vi "SNEdit.vi"() -> ()   [LabVIEW 2011]
uses:
  data/VCI_CAN.dll
panel:
  in  "devtype":u16(ring)=2 caption="设备类型：" items=["USB-CAN"=2, "USB-CAN2.0"=3]
  in  "snedit":bool
  in  "close":bool
  in  "open":bool
  out "canopen":bool caption="设备打开："
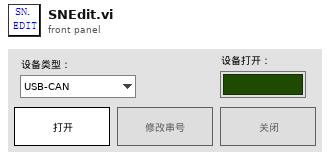
[diagram p1: front panel]
types:
  T1 = enum16{"Init", "EventReg", "Run", "Release", "Exit"}
  T2 = cluster{"hw_Version":u16, "fw_Version":u16, "dr_Version":u16, "in_Version":u16, "irq_Num":u16, "can_Num":u8, "str_Serial_Num":string, "str_hw_Type":string, "Reserved":u8[]}
  T3 = cluster{"hw_Version":u16, "fw_Version":u16, "dr_Version":u16, "in_Version":u16, "irq_Num":u16, "can_Num":u8, "reserved":u8, "str_Serial_Num":string, "str_hw_Type":string, "str_GYUsb_Serial":string[]}
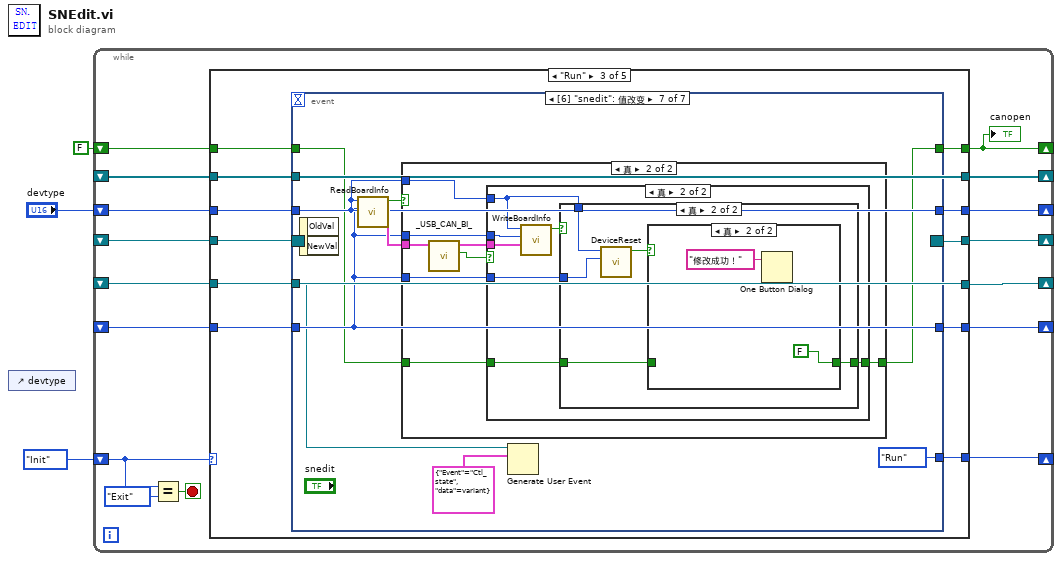
[diagram p0: block diagram]
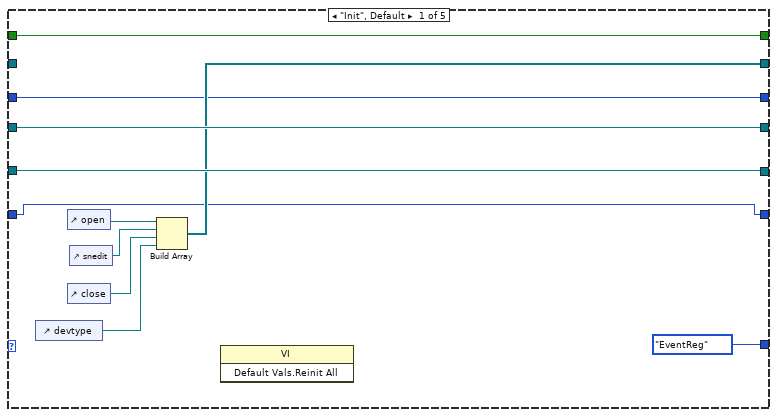
[diagram p2: hidden frame]
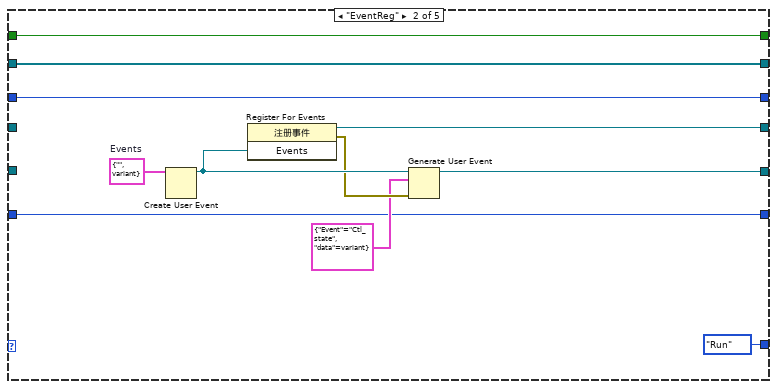
[diagram p3: hidden frame]
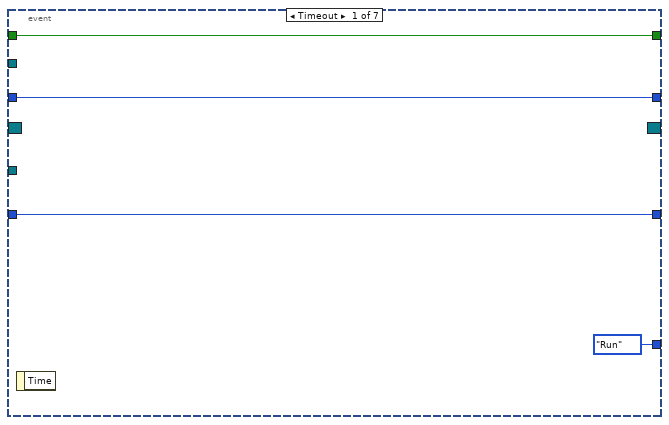
[diagram p4: hidden frame]
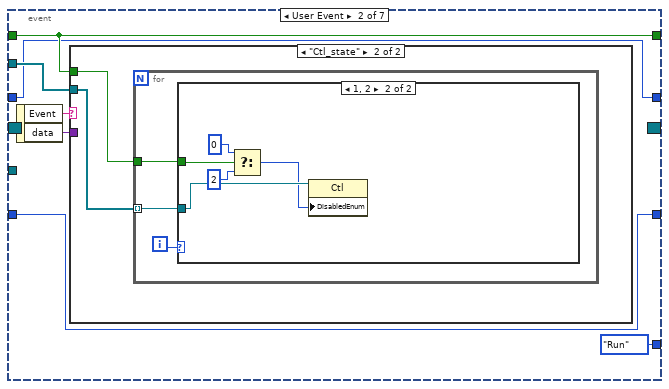
[diagram p5: hidden frame]
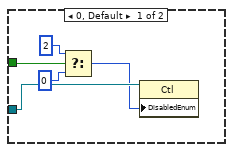
[diagram p7: hidden frame]
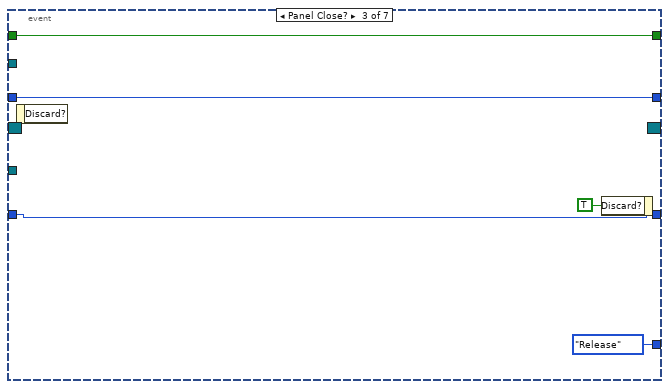
[diagram p8: hidden frame]
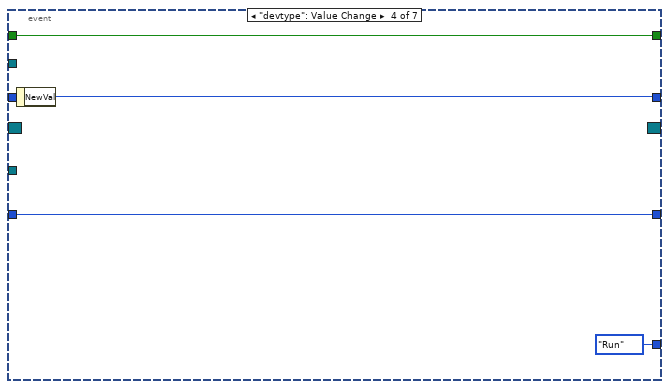
[diagram p9: hidden frame]
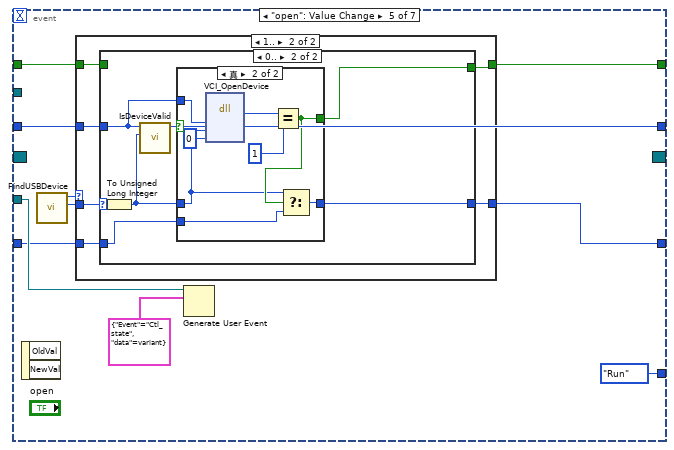
[diagram p10: hidden frame]
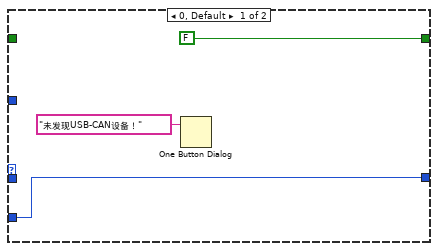
[diagram p11: hidden frame]
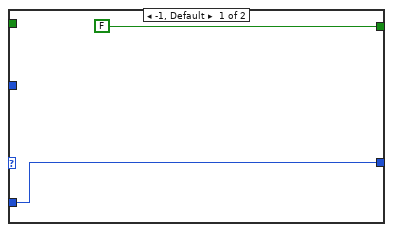
[diagram p12: hidden frame]
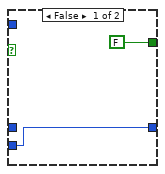
[diagram p13: hidden frame]
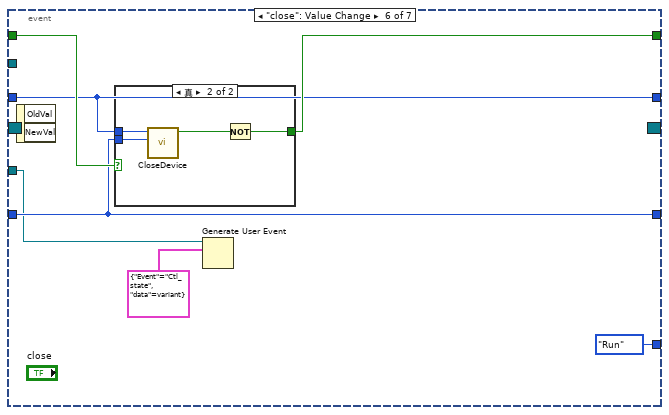
[diagram p14: hidden frame]
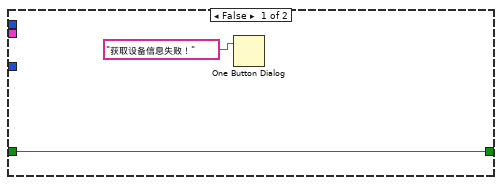
[diagram p16: hidden frame]
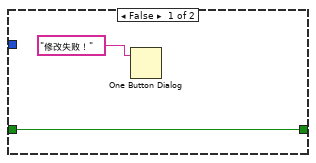
[diagram p18: hidden frame]
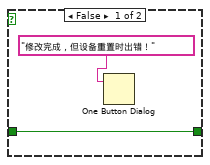
[diagram p19: hidden frame]
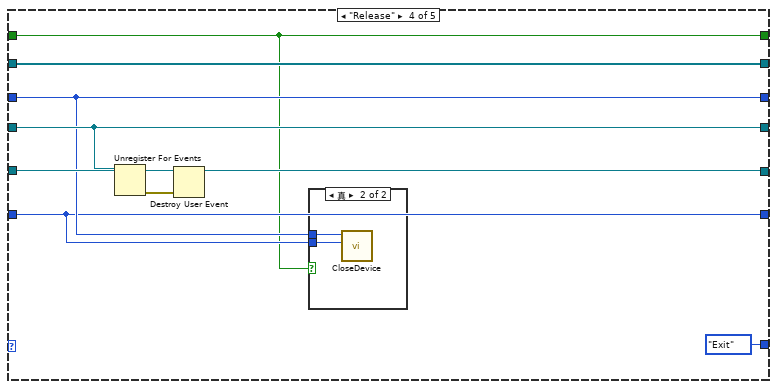
[diagram p20: hidden frame]
diagram:
  n1 = control-ref of="devtype"() -> ()  [unwired: 1 out]
  n2 = while {
    shift-right: [w16] -> _
    shift-left: T1."Init" -> [w19]
    shift-right: [w8] -> _
    shift-left: FALSE -> [w15]
    shift-right: [w14] -> _
    shift-left: _ -> [w13]
    shift-right: [w12] -> _
    shift-left: _ -> [w11]
    shift-right: [w10] -> _
    shift-left: _ -> [w9]
    shift-right: [w6] -> _
    shift-left: "devtype" -> [w7]
    shift-right: [w5] -> _
    shift-left: _ -> [w4]
    stop <- w18 stop-if-true
    n3 = Equal?(x=w19, y=T1."Exit") -> (x = y?=w18:bool)
    n4 = case shown="\"Run\"" w19 {
      tunnel: [T1."EventReg" T1."Run" w48 T1."Exit" T1."Exit"] -> w16
      tunnel: w15 -> [w29 w40 w52 w176 w193]
      tunnel: [w29 w40 w51 w176 w193] -> w8
      tunnel: [w28 w36 w49 w182 w192] -> w14
      tunnel: w13 -> [w28 _ w50 w182 w192]
      tunnel: [w27 w35 w46 w180 w191] -> w12
      tunnel: w11 -> [w27 _ w46 w180 w191]
      tunnel: [w23 w33 w47 w179 w189] -> w10
      tunnel: w9 -> [_ w33 w47 w179 w189]
      tunnel: w7 -> [w22 w32 w45 w178 w188]
      tunnel: [w22 w32 w44 w178 w188] -> w6
      tunnel: [w21 w31 w43 w177 w187] -> w5
      tunnel: w4 -> [w21 w31 w42 w177 w187]
      frame "Init", Default {
        n5 = control-ref of="devtype"() -> (w20:refnum<vi>)
        n6 = control-ref of="open"() -> (w26:refnum<vi>)
        n7 = control-ref of="close"() -> (w24:refnum<vi>)
        n8 = control-ref of="snedit"() -> (w25:refnum<vi>)
        n9 = Build Array(w26, w25, w24, w20) -> (w23:refnum<vi>[])
        n10 = invoke class="VI" method="Default Vals.Reinit All"() -> ()  [unwired: 3 in, 3 out]
      }
      frame "EventReg" {
        w39 = cluster{"Event":string, "data":variant} {"Event"="", "data"=variant}  # Events
        n11 = Create User Event(user event datatype=w39) -> (user event=w38:refnum<user-event>)  [unwired: 1 in, 1 out]
        n12 = register-events(w38) -> (reference out=w36:refnum<event-registration>, error out=w37:errorcluster)  [unwired: 2 in]
        n13 = Generate User Event(user event=w38, event data cluster=cluster{"Event":string, "data":variant} {"Event"="Ctl_state", "data"=variant} ("事件数据"), error in=w37) -> (user event out=w35:refnum<user-event>)  [unwired: 1 out]
      }
      frame "Run" {
        n14 = event shown="[6] \"snedit\": 值改变" {
          selector: w50 -> [_ _ _ _ _ _ _]
          dyn-events: [_ _ _ _ _ _ _] -> w49
          timeout: _ -> [_ _ _ _ _ _ _]
          tunnel: w52 -> [w56 w59 w81 w87 w96 w131 w141]
          tunnel: [w56 w59 w81 w87 w94 w130 w140] -> w51
          tunnel: [T1."Run" T1."Run" T1."Release" T1."Run" T1."Run" T1."Run" T1."Run"] -> w48
          tunnel: w47 -> [_ w60 _ _ _ _ _]
          tunnel: w45 -> [w54 w58 w80 _ w90 w129 w143]
          tunnel: w46 -> [_ _ _ _ w92 w126 w138]
          tunnel: [w54 w58 w80 w86 w90 w129 w143] -> w44
          tunnel: [w53 w57 w79 w84 w89 w128 w142] -> w43
          tunnel: w42 -> [w53 w57 w79 w84 w88 w128 w142]
          event Timeout {
            n15 = event-data() -> ()  [unwired: 1 in, 1 out]
          }
          event User Event {
            n16 = event-data() -> ("Event"=w62:string, "data"=w61:variant)  [unwired: 1 in]
            n17 = case shown="\"Ctl_state\"" w62 {
              tunnel: w61 -> [_ _]
              tunnel: w60 -> [_ w65]
              tunnel: w59 -> [_ w64]
              frame "假", Default {
              }
              frame "Ctl_state" {
                n18 = for {
                  tunnel: w65 -> [w66] mode=indexing
                  tunnel: w64 -> [w67]
                  i -> [w68]
                  n19 = case shown="1, 2" w68 {
                    tunnel: w67 -> [w72 w77]
                    tunnel: w66 -> [w73 w78]
                    frame 0, Default {
                      n20 = Select(t=2, s=w72, f=0) -> (s? t:f=w69:i32)
                      n21 = property class="Ctl"(reference=w73, "DisabledEnum"=w69) -> ()  [unwired: 1 in, 2 out]
                    }
                    frame 1, 2 {
                      n22 = Select(t=0, s=w77, f=2) -> (s? t:f=w74:i32)
                      n23 = property class="Ctl"(reference=w78, "DisabledEnum"=w74) -> ()  [unwired: 1 in, 2 out]
                    }
                  }
                }
              }
            }
          }
          event Panel Close? {
            n24 = event-data() -> ()  [unwired: 1 in, 1 out]
            n25 = event-data("Discard?"=TRUE ("放弃？")) -> ()  [unwired: 1 in, 1 out]
          }
          event "devtype": Value Change {
            n26 = event-data() -> ("NewVal"=w86:u16)  [unwired: 1 in]
          }
          event "open": Value Change {
            n27 = event-data() -> ()  [unwired: 1 in, 2 out]
            n28 = call "FindUSBDevice.vi"() -> ("DevNum"=w93:i32, "Total"=w95:u32)  [unwired: 7 in, 3 out]
            n29 = case shown="1.." w95 {
              tunnel: w96 -> [_ w105]
              tunnel: [FALSE w104] -> w94
              tunnel: w93 -> [_ w106]
              tunnel: w90 -> [_ w103]
              tunnel: [w98 w102] -> w89
              tunnel: w88 -> [w98 w101]
              frame 0, Default {
                n30 = One Button Dialog(message="未发现USB-CAN设备！" ("消息")) -> ()  [unwired: 1 in, 1 out]
              }
              frame 1.. {
                n31 = case shown="0.." w106 {
                  selector: w106 -> [_ w115]
                  tunnel: w105 -> [_ _]
                  tunnel: [FALSE w111] -> w104
                  tunnel: w103 -> [_ w113]
                  tunnel: [w107 w110] -> w102
                  tunnel: w101 -> [w107 w109]
                  frame -1, Default {
                  }
                  frame 0.. {
                    n32 = To Unsigned Long Integer(number=w115) -> (unsigned 32bit integer=w112:u32)
                    n33 = call "IsDeviceValid.vi"("DeviceInd"=w112, "type"=w113) -> ("Valid"=w114:bool)  [unwired: 8 in, 1 out]
                    n34 = case shown="真" w114 {
                      tunnel: w113 -> [_ w125]
                      tunnel: w112 -> [_ w120]
                      tunnel: [FALSE w121] -> w111
                      tunnel: [w116 w118] -> w110
                      tunnel: w109 -> [w116 w119]
                      frame False {
                      }
                      frame True {
                        n35 = dll-call lib="PTH1Kabs D\t董海成\t上位机2.进行中USB-CAN TooldataVCI_CAN.dll" fn="VCI_OpenDevice"("DevType"=w125, "DevIndex"=w120, "Reserved"=u32 0) -> ("返回类型"=w123:u32)  [unwired: 6 in, 2 out]
                        n36 = Equal?(x=w123, y=u32 1) -> (x = y?=w121:bool)
                        n37 = Select(t=w120, s=w121, f=w119) -> (s? t:f=w118:u32)
                      }
                    }
                  }
                }
              }
            }
            n38 = Generate User Event(user event=w92, event data cluster=cluster{"Event":string, "data":variant} {"Event"="Ctl_state", "data"=variant} ("事件数据")) -> ()  [unwired: 1 in, 2 out]
          }
          event "close": Value Change {
            n39 = event-data() -> ()  [unwired: 1 in, 2 out]
            n40 = case shown="真" w131 {
              selector: w131 -> [w133 _]
              tunnel: w129 -> [_ w137]
              tunnel: w128 -> [_ w136]
              tunnel: [w133 w134] -> w130
              frame False {
              }
              frame True {
                n41 = call "CloseDevice.vi"("DeviceInd"=w136, "type"=w137) -> ("success"=w135:bool)  [unwired: 8 in, 1 out]
                n42 = Not(x=w135) -> (.not. x?=w134:bool)
              }
            }
            n43 = Generate User Event(user event=w126, event data cluster=cluster{"Event":string, "data":variant} {"Event"="Ctl_state", "data"=variant} ("事件数据")) -> ()  [unwired: 1 in, 2 out]
          }
          event "snedit": Value Change {
            n44 = event-data() -> ()  [unwired: 1 in, 2 out]
            n45 = call "ReadBoardInfo.vi"("DeviceInd"=w142, "DeviceType"=w143) -> ("VCI_BOARD_INFO"=w145:T2, "success"=w144:bool)  [unwired: 8 in]
            n46 = case shown="真" w144 {
              tunnel: w145 -> [_ w156]
              tunnel: w143 -> [_ w153]
              tunnel: w142 -> [_ w152]
              tunnel: w142 -> [_ w151]
              tunnel: w141 -> [w148 w150]
              tunnel: [w148 w149] -> w140
              frame False {
                n47 = One Button Dialog(message="获取设备信息失败！" ("Infoin")) -> ()  [unwired: 1 in, 1 out]
              }
              frame True {
                n48 = call "_USB_CAN_BI_.vi"("BOARD_INFO"=w156) -> ("change?"=w155:bool, "BOARD_INFO out"=w154:T3)  [unwired: 9 in]
                n49 = case shown="真" w155 {
                  tunnel: w154 -> [_ w164]
                  tunnel: w153 -> [_ w161]
                  tunnel: w152 -> [_ w163]
                  tunnel: w151 -> [_ w160]
                  tunnel: w150 -> [w157 w159]
                  tunnel: [w157 w158] -> w149
                  frame False {
                  }
                  frame True {
                    n50 = call "WriteBoardInfo.vi"("BOARD_INFO"=w164, "DeviceInd"=w163, "DeviceType"=w161) -> ("success"=w162:bool)  [unwired: 8 in]
                    n51 = case shown="真" w162 {
                      tunnel: w161 -> [_ w171]
                      tunnel: w160 -> [_ w170]
                      tunnel: w159 -> [w166 w168]
                      tunnel: [w166 w167] -> w158
                      frame False {
                        n52 = One Button Dialog(message="修改失败！" ("Infoin")) -> ()  [unwired: 1 in, 1 out]
                      }
                      frame True {
                        n53 = call "DeviceReset.vi"("DeviceInd"=w170, "DeviceType"=w171) -> ("Success"=w169:bool)  [unwired: 9 in]
                        n54 = case shown="真" w169 {
                          tunnel: w168 -> [w172 _]
                          tunnel: [w172 FALSE] -> w167
                          frame False {
                            n55 = One Button Dialog(message="修改完成，但设备重置时出错！" ("Infoin")) -> ()  [unwired: 1 in, 1 out]
                          }
                          frame True {
                            n56 = One Button Dialog(message="修改成功！" ("Infoin")) -> ()  [unwired: 1 in, 1 out]
                          }
                        }
                      }
                    }
                  }
                }
              }
            }
            n57 = Generate User Event(user event=w138, event data cluster=cluster{"Event":string, "data":variant} {"Event"="Ctl_state", "data"=variant} ("事件数据")) -> ()  [unwired: 1 in, 2 out]
          }
        }
      }
      frame "Release" {
        n58 = Unregister For Events(event registration refnum=w182) -> (error out=w181:errorcluster)  [unwired: 1 in]
        n59 = Destroy User Event(user event=w180, error in=w181) -> ()  [unwired: 1 out]
        n60 = case shown="真" w176 {
          tunnel: w178 -> [_ w185]
          tunnel: w177 -> [_ w184]
          frame False {
          }
          frame True {
            n61 = call "CloseDevice.vi"("DeviceInd"=w184, "type"=w185) -> ()  [unwired: 8 in, 2 out]
          }
        }
      }
      frame "Exit" {
        n62 = control-ref of="本VI"() -> (w186:refnum<vi>)
        n63 = call "Exit.vi"("VI引用"=w186) -> ()  [unwired: 10 in, 1 out]
      }
    }
    "canopen" <- w8
  }
